vi "Smooth lifting.vi"(9 "Lifting rotation":i32=550, 11 "EV3 in":T1) -> (3 "EV3 out":T1)   [LabVIEW 2016]
uses:
  <vilib>/NXT/Subs/LVHSConnector.ctl
  <vilib>/NXT/LegoClasses/BrickReference/BrickReference.lvclass
  <vilib>/NXT/Block Support/NXT_OutputPort.ctl
  <vilib>/NXT/NXTIO Xnodes/NXTIONodeSubVIs/LEGOResetMotors.vi
  <vilib>/NXT/Dual Mode Library/Motors/Rotation.vi
  <vilib>/NXT/NXTIO Xnodes/NXTIONodeSubVIs/NXTMoveMotors.vi
  <vilib>/NXT/NXTIO Xnodes/NXTIONodeSubVIs/NXTStopMotors.vi
  <vilib>/NXT/Dual Mode Library/Waits/Wait_Num.vi
  <vilib>/NXT/NXTIO Xnodes/NXTIOXNode/NXTIO.xnode
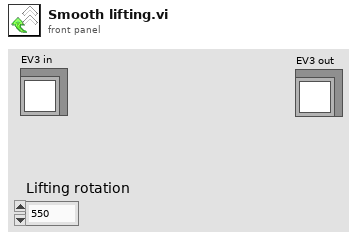
[diagram p1: front panel]
types:
  T1 = typedef "LVHSConnector.ctl" = refnum<class "BrickReference.lvclass">
  T2 = typedef "NXT_OutputPort.ctl" = u8
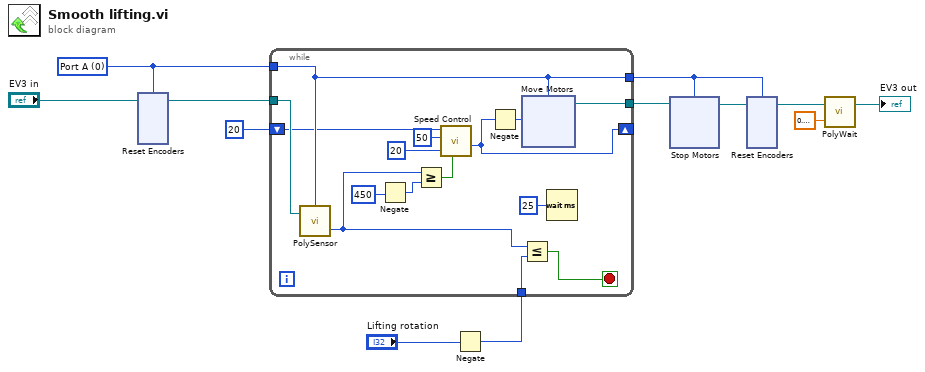
[diagram p0: block diagram]
diagram:
  w4 = T2 0 items=["Port A", "Port B", "Port C", "Port D"] ("Port (Port A)")
  n1 = xnode "Reset Encoders"("Motors"=w4, "NXT/EV3"="EV3 in") -> ("NXT/EV3"=w5:T1)
  n2 = Negate(x="Lifting rotation") -> (-x=w1:i32)
  n3 = while {
    tunnel: [w24] -> w11
    tunnel: w5 -> [w26]
    tunnel: [w23] -> w6
    tunnel: w4 -> [w23]
    shift-right: [w15] -> _
    shift-left: 20 ("Min. speed") -> [w18]
    tunnel: w1 -> [w13]
    stop <- w27 stop-if-true
    n4 = call-poly <vilib>:"PolySensor.vi"("NXT/EV3"=w26, "Port (Port A)"=w23) -> ("Angle of Rotation"=w21:i32)  [unwired: 1 in, 1 out]
    n5 = Negate(x=450 ("y")) -> (-x=w14:i32)
    n6 = Greater Or Equal?(x=w21, y=w14) -> (x >= y?=w19:bool)
    n7 = call "Speed Control.vi"("Speed Up or Down?"=w19, "Min. speed"=20, "Max. speed"=50, "Ini. speed"=w18) -> ("Speed out"=w15:i32)  [unwired: 7 in]
    n8 = Negate(x=w15) -> (-x=w25:i32)
    n9 = xnode "Move Motors"("Power/Speed 1"=w25, "Motors"=w23) -> ("NXT/EV3"=w24:T1)  [unwired: 1 in]
    n10 = Less Or Equal?(x=w21, y=w13) -> (x <= y?=w27:bool)
    n11 = Wait (ms)(milliseconds to wait=u32 25) -> ()  [unwired: 1 out]
  }
  n12 = xnode "Stop Motors"("Motors"=w6, "NXT/EV3"=w11) -> ("NXT/EV3"=w10:T1)
  n13 = xnode "Reset Encoders"("Motors"=w6, "NXT/EV3"=w10) -> ("NXT/EV3"=w8:T1)
  n14 = call-poly <vilib>:"PolyWait.vi"("Time (1 sec)"=sgl 0.2, "NXT/EV3"=w8) -> ("NXT/EV3"=→"EV3 out":T1)  [unwired: 2 in]
